vi "my Normalize(子VI).vi"(1 "N-1":i32, 2 "Data":dbl[][](array[numeric])) -> (0 "Normlized":dbl[][](array[numeric]))   [LabVIEW 2018]
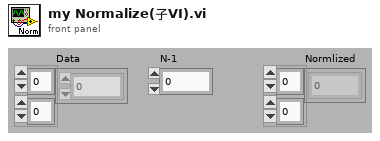
[diagram p1: front panel]
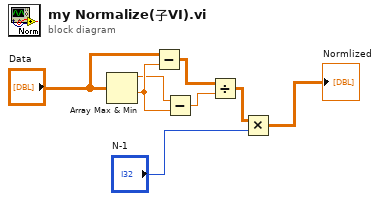
[diagram p0: block diagram]
diagram:
  n1 = Array Max & Min(array="Data") -> (max value=w1:dbl, min value=w2:dbl)  [unwired: 2 out]
  n2 = Subtract(x="Data", y=w2) -> (x-y=w3:dbl[][])
  n3 = Subtract(x=w1, y=w2) -> (x-y=w4:dbl)
  n4 = Divide(x=w3, y=w4) -> (x/y=w6:dbl[][])
  n5 = Multiply(x=w6, y="N-1") -> (x*y=→"Normlized":dbl[][])
